vi "Configure IQ vs Slot Measurement List.vi"(6 "Expected Nominal Powers":dbl[](array[numeric]) format="%.2p", 7 "Frequencies":dbl[](array[numeric]) format="%.2p", 8 "error in (no error)":errorcluster, 9 "List Length (10)":i32=10, 10 "Instance (1)":i32=1 format="%.0g", 11 "VISA resource name":refnum<visa-resource-name>) -> (0 "error out":errorcluster, 3 "VISA resource name out":refnum<visa-resource-name>)   [LabVIEW 2015, in "Rohde&Schwarz CMXP GPRF.lvlib"]
doc: "Configures list of IQ vs Slot measurement points.\n\nAttributes:\nRSCMXPGPRF_ATTR_SET_IQ_VS_SLOT_MEASUREMENT_LIST_STEP_FREQUENCY\nRSCMXPGPRF_ATTR_SET_IQ_VS_SLOT_MEASUREMENT_LIST_STEP_EXPECTED_NOMINAL_POWER\n\nRemote-control commands:\nCONFigure:GPRF:MEAS<i>:IQVSlot:LIST:FREQuency:ALL\nCONFigure:GPRF:MEAS<i>:IQVSlot:LIST:ENPower:ALL"
uses:
  <instrlib>/Rohde&Schwarz CMXP GPRF/Rohde&Schwarz CMXP GPRF.lvlib
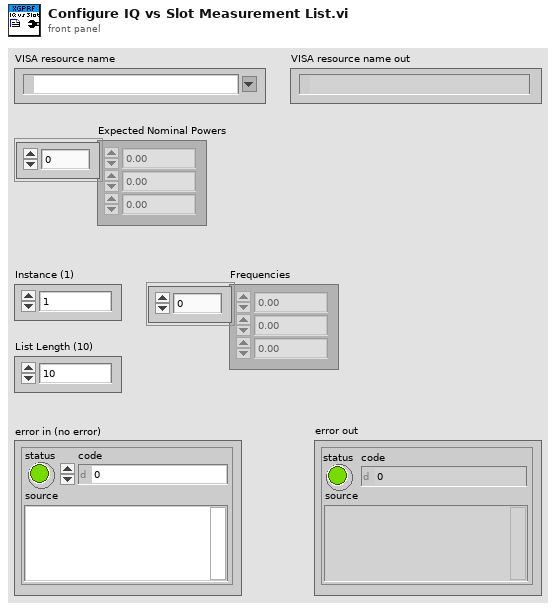
[diagram p1: front panel]
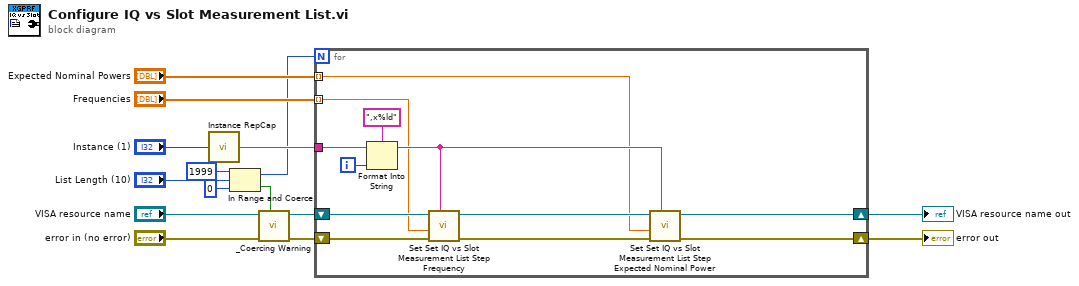
[diagram p0: block diagram]
diagram:
  n1 = call <instrlib>:"Instance RepCap.vi"("instance  in"="Instance (1)") -> ("instance out"=w10:string)
  n2 = In Range and Coerce(upper limit=1999, x="List Length (10)", lower limit=0) -> (coerced(x)=w1:i32, In Range?=w12:bool)
  n3 = call <instrlib>:"_Coercing Warning.vi"("In Range?"=w12, "error in (no error)"="error in (no error)", "VISA resource name"="VISA resource name") -> ("error out"=w14:errorcluster, "VISA resource name out"=w13:refnum<visa-resource-name>)  [unwired: 7 in]
  n4 = for {
    N: w1 -> [_]
    tunnel: w10 -> [w18]
    shift-right: [w22] -> w8
    shift-left: w14 -> [w23]
    tunnel: "Frequencies" -> [w17] mode=indexing
    tunnel: "Expected Nominal Powers" -> [w16] mode=indexing
    shift-right: [w25] -> w9
    shift-left: w13 -> [w24]
    i -> [w21]
    n5 = Format Into String(format string=",x%ld", initial string=w18, w21) -> (resulting string=w19:string)  [unwired: 1 in, 1 out]
    n6 = call "Set Set IQ vs Slot Measurement List Step Frequency"("Repeated Capabilities"=w19, "error in (no error)"=w23, "Set IQ vs Slot Measurement List Step Frequency (0.0)"=w17, "instrument handle"=w24) -> ("error out"=w26:errorcluster, "instrument handle out"=w27:refnum<visa-resource-name>)  [unwired: 6 in]
    n7 = call "Set Set IQ vs Slot Measurement List Step Expected Nominal Power"("Repeated Capabilities"=w19, "error in (no error)"=w26, "Set IQ vs Slot Measurement List Step Expected Nominal Power (0.0)"=w16, "instrument handle"=w27) -> ("error out"=w22:errorcluster, "instrument handle out"=w25:refnum<visa-resource-name>)  [unwired: 6 in]
  }
  "error out" <- w8
  "VISA resource name out" <- w9
